vi "Remove-inactive-client.vi"(8 "error in (no error)":errorcluster, 10 "Client index":i32, 11 "ModComm in":T1) -> (0 "error out":errorcluster, 3 "ModComm out":T1)   [LabVIEW 2013, in "SLMServer.lvlib" / "SLMServer.lvclass"]
uses:
  SLMServer.lvclass
  Object-reference.ctl
  UI-messages.ctl
  SLMServer.lvclass/SLMServer.ctl
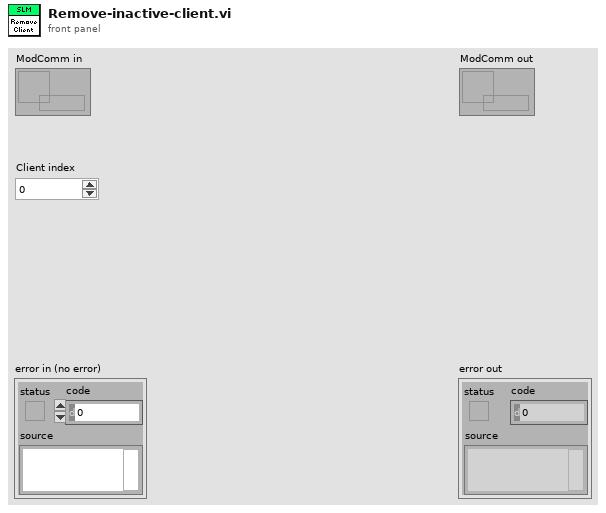
[diagram p1: front panel]
types:
  T1 = typedef "SLMServer.lvlib/SLMServer.lvclass/Object-reference.ctl" = refnum<data-value>
  T2 = typedef "SLMServer.lvlib/SLMServer.lvclass/UI-messages.ctl" = enum16{"Time out", "User cancel", "Module cancel", "Client inactivity", "Client limit", "Client started"}
  T3 = typedef "SLMServer.lvlib/SLMServer.lvclass/Supported-module-types.ctl" = enum16{"SLMControl", "PowderDeposition", "CameraVision", "Server", "All", "StrategyParser", "MaterialCharacterization", "StatusMonitor", "SLMSimulation", "LaserCharacterization"}
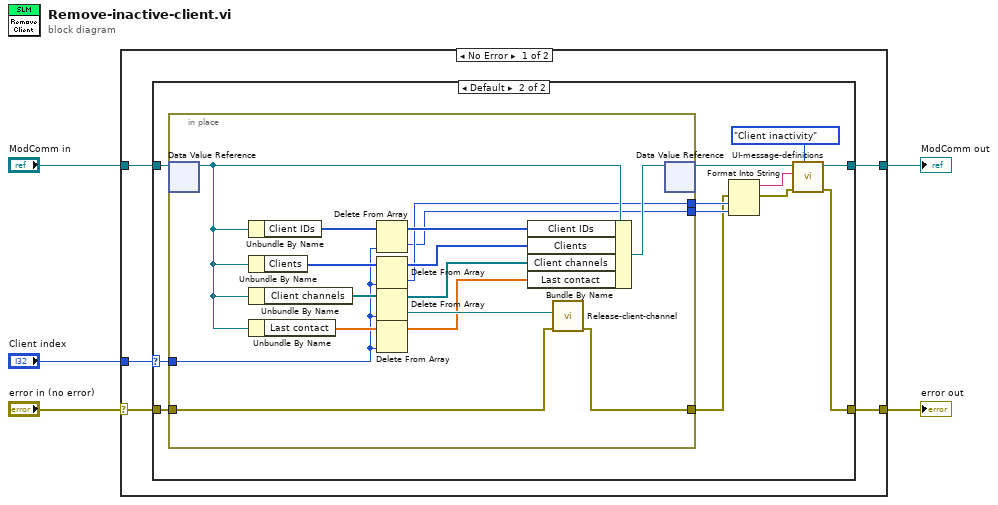
[diagram p0: block diagram]
diagram:
  n1 = case shown="No Error" "error in (no error)" {
    selector: "error in (no error)" -> [w9 w42]
    tunnel: [w7 w42] -> w4
    tunnel: [w8 w41] -> w2
    tunnel: "ModComm in" -> [w10 w41]
    tunnel: "Client index" -> [w6 _]
    frame No Error {
      n2 = case shown="Default" w6 {
        selector: w6 -> [_ w13]
        tunnel: w10 -> [w11 w24]
        tunnel: w9 -> [w12 w23]
        tunnel: [w11 w21] -> w8
        tunnel: [w12 w20] -> w7
        frame -1 {
        }
        frame Default {
          n3 = in-place {
            in-place-border: w13 -> [w36]
            in-place-border: w23 -> [w34]
            in-place-border: [w27] -> w16
            in-place-border: [w26] -> w19
            in-place-border: [w25] -> w18
            n4 = in-place-dvr #1(w24) -> (w28:refnum<class "SLMServer.lvclass">)  [unwired: 1 out]
            n5 = Unbundle By Name(w28) -> ("Client IDs"=w40:i32[])
            n6 = Unbundle By Name(w28) -> ("Clients"=w39:T3[])
            n7 = Unbundle By Name(w28) -> ("Client channels"=w38:refnum<queue>[])
            n8 = Unbundle By Name(w28) -> ("Last contact"=w37:dbl[])
            n9 = Delete From Array(array=w40, index=w36) -> (deleted portion=w25:i32, array with subset deleted=w33:i32[])  [unwired: 1 in]
            n10 = Delete From Array(array=w39, index=w36) -> (deleted portion=w26:T3, array with subset deleted=w32:T3[])  [unwired: 1 in]
            n11 = Delete From Array(array=w38, index=w36) -> (deleted portion=w35:refnum<queue>, array with subset deleted=w31:refnum<queue>[])  [unwired: 1 in]
            n12 = Delete From Array(array=w37, index=w36) -> (array with subset deleted=w30:dbl[])  [unwired: 1 in, 1 out]
            n13 = Bundle By Name(cluster=w28, "Client IDs"=w33, "Clients"=w32, "Client channels"=w31, "Last contact"=w30) -> (w29:refnum<class "SLMServer.lvclass">)
            n14 = call "Release-client-channel.vi"("error in (no error)"=w34, "Comm channel"=w35) -> ("error out"=w27:errorcluster)  [unwired: 9 in]
            n15 = in-place-dvr #1(w29) -> (w22:T1)  [unwired: 1 out]
          }
          n16 = Format Into String(error in=w16, w19, w18) -> (resulting string=w14:string, error out=w17:errorcluster)  [unwired: 2 in]
          n17 = call "UI-message-definitions.vi"("Message"=UI-messages."Client inactivity", "error in (no error)"=w17, "Additional text"=w14, "ModComm in"=w22) -> ("error out"=w20:errorcluster, "ModComm out"=w21:T1)  [unwired: 6 in]
        }
      }
    }
    frame Error {
    }
  }
  "error out" <- w4
  "ModComm out" <- w2
